vi "Configure Trigger Coupling.vi"(8 "error in (no error)":errorcluster, 10 "Coupling Channel (0: None)":i32(ring) items=["None", "All", "Channel 1 And 2", "Channel 1 And 3", "Channel 2 And 3"], 11 "VISA resource name":refnum<visa-resource-name>) -> (0 "error out":errorcluster, 3 "VISA resource name out":refnum<visa-resource-name>)   [LabVIEW 2020, in "Keysight E36300 Series.lvlib"]
doc: "Configures a defined coupling between various logical outputs of the power supply. Coupled outputs will be triggered simultaneously once a trigger is sent.\n\n<b>Note:</b> \nThis VI is only applicable for E3631A personal mode."
uses:
  Keysight E36300 Series.lvlib
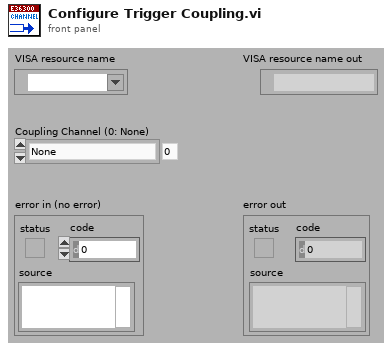
[diagram p1: front panel]
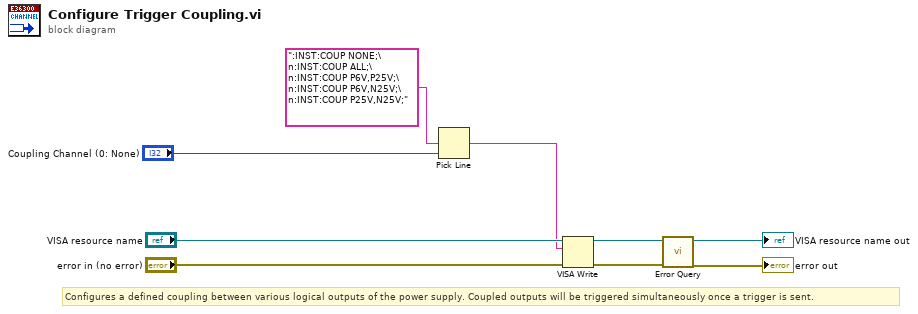
[diagram p0: block diagram]
diagram:
  # "Configures a defined coupling between various logical outputs of the power supply. Coupled outputs will be triggered simultaneously once a trigger is sent."
  n1 = Pick Line(multi-line string=":INST:COUP NONE;\n:INST:COUP ALL;\n:INST:COUP P6V,P25V;\n:INST:COUP P6V,N25V;\n:INST:COUP P25V,N25V;", line index="Coupling Channel (0: None)") -> (output string=w1:string)  [unwired: 1 in]
  n2 = VISA Write(VISA resource name="VISA resource name", write buffer=w1, error in (no error)="error in (no error)") -> (VISA resource name out=w7:refnum<visa-resource-name>, error out=w6:errorcluster)  [unwired: 1 out]
  n3 = call "Error Query.vi"("error in (no error)"=w6, "VISA resource name"=w7) -> ("error out"=→"error out":errorcluster, "VISA resource name out"=→"VISA resource name out":refnum<visa-resource-name>)  [unwired: 6 in, 2 out]
